vi "Contains.vi"(8 "error in (no error)":errorcluster, 10 "Key":string, 11 "VariantAttribute in":refnum<class "MapImp.lvclass">) -> (0 "error out":errorcluster, 1 "Key Exists?":bool, 3 "VariantAttribute out":refnum<class "MapImp.lvclass">)   [LabVIEW 2013, in "LapDog.Collections.v_.Maps.lvlib" / "MapImp.lvclass"]
doc: "Returns a boolean True if the key exists in the map."
uses:
  MapImp.lvclass
  MapImp.lvclass/MapImp.ctl
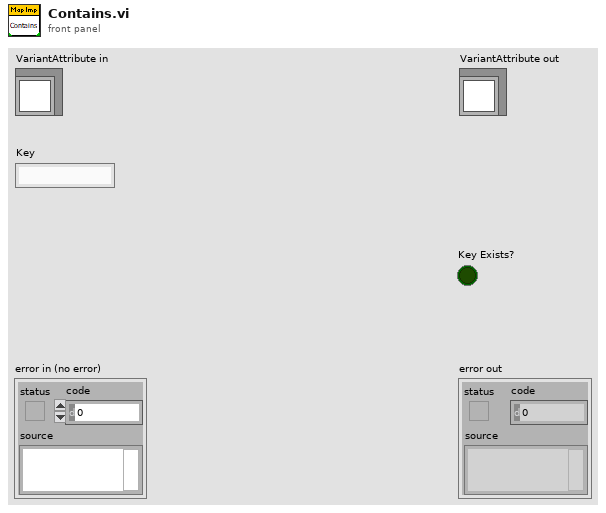
[diagram p1: front panel]
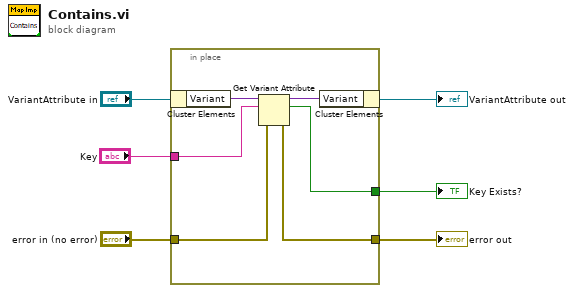
[diagram p0: block diagram]
diagram:
  n1 = in-place {
    in-place-border: "Key" -> [w10]
    in-place-border: [w9] -> w4
    in-place-border: "error in (no error)" -> [w8]
    in-place-border: [w7] -> w1
    n2 = in-place-cluster #1("VariantAttribute in") -> ("Variant"=w12:variant)
    n3 = Get Variant Attribute(Variant=w12, name=w10, error in=w8) -> (duplicate Variant=w11:variant, found=w9:bool, error out=w7:errorcluster)  [unwired: 1 in, 1 out]
    n4 = in-place-cluster #1("Variant"=w11) -> (→"VariantAttribute out":refnum<class "MapImp.lvclass">)
  }
  "error out" <- w1
  "Key Exists?" <- w4
